vi "Joystick Driver Controls_Timmer.vi"(7 "X":dbl, 11 "Y":dbl) -> (2 "Y":dbl, 3 "X":dbl)   [LabVIEW 2017]
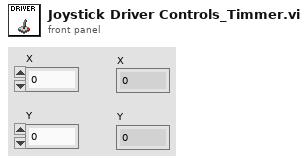
[diagram p1: front panel]
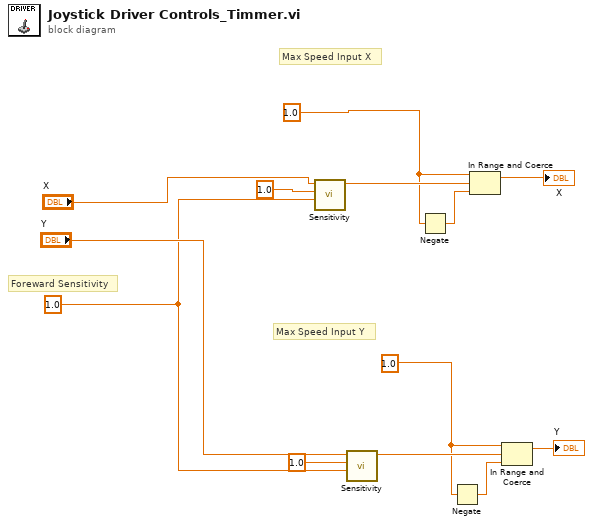
[diagram p0: block diagram]
diagram:
  w2 = 1.0 ("x")
  w3 = 1.0 ("Default Value")
  w1 = 1.0 ("Default Value")
  # "Foreward Sensitivity"
  # "Max Speed Input Y"
  # "Max Speed Input X"
  n1 = call "Sensitivity.vi"("Power (z)"=w1, "Sensitivity (a)"=1.0, "Input"="X") -> ("Output"=w7:dbl)  [unwired: 8 in]
  n2 = call "Sensitivity.vi"("Power (z)"=w1, "Sensitivity (a)"=1.0, "Input"="Y") -> ("Output"=w11:dbl)  [unwired: 8 in]
  n3 = Negate(x=w3) -> (-x=w8:dbl)
  n4 = Negate(x=w2) -> (-x=w13:dbl)
  n5 = In Range and Coerce(upper limit=w3, x=w7, lower limit=w8) -> (coerced(x)=→"X":dbl)  [unwired: 1 out]
  n6 = In Range and Coerce(upper limit=w2, x=w11, lower limit=w13) -> (coerced(x)=→"Y":dbl)  [unwired: 1 out]
